vi "Undersample_NB.vi"(6 "error in (no error)":errorcluster, 7 "Unit Info":string="Unit1", 8 "U/S Frequency":i32=2400, 9 "U/S Location":string(combo)="VCO") -> (0 "error out":errorcluster, 2 "Cycle-Cycle Jitter":string, 3 "Total RMS Jitter":string)   [LabVIEW 2011]
doc: "This VI undersamples a selected signal from the NB PLL at a specified frequency.\n\nInputs:\n1. U/S Location: Part of PLL loop to be undersamles (VCO, PllOut, VCO_Z, Spine, etc).\n2. U/S Frequency: Frequency at which the PLL to be undersampled is running (2400, 2600, etc.)\n3. Unit Info: Information about the unit to attach to undersampling results file.\n\nOutputs:\n1. Total RMS Jitter: The total RMS Jitter as read from the resultspectrum file.\n2. Cycle-Cycle Jitter: The Cycle-Cycle Jitter as read from the result spectrum file."
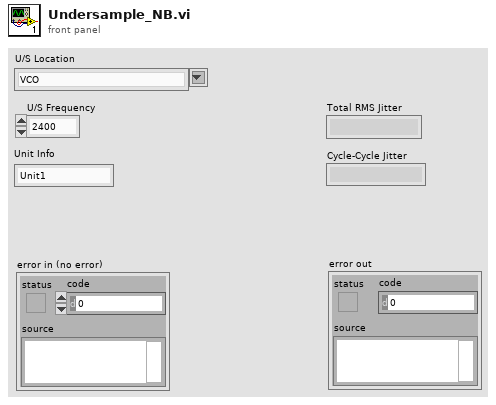
[diagram p1: front panel]
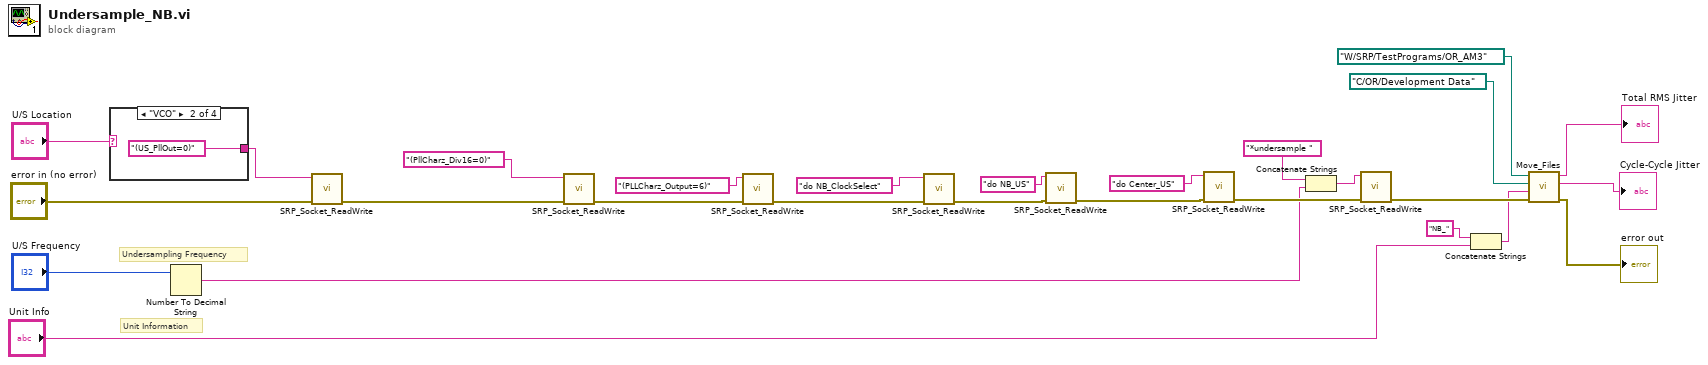
[diagram p0: block diagram]
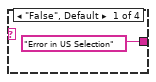
[diagram p2: hidden frame]
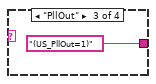
[diagram p3: hidden frame]
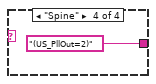
[diagram p4: hidden frame]
diagram:
  # "Unit Information"
  # "Undersampling Frequency"
  n1 = case shown="\"VCO\"" "U/S Location" {
    tunnel: ["Error in US Selection" "(US_PllOut=0)" "(US_PllOut=1)" "(US_PllOut=2)"] -> w10
    frame "False", Default {
    }
    frame "VCO" {
    }
    frame "PllOut" {
    }
    frame "Spine" {
    }
  }
  n2 = Number To Decimal String(number="U/S Frequency") -> (decimal integer string=w2:string)  [unwired: 1 in]
  n3 = call "SRP_Socket_ReadWrite.vi"("error in (no error)"="error in (no error)", "Data In"=w10) -> ("error out"=w24:errorcluster)  [unwired: 7 in, 1 out]
  n4 = call "SRP_Socket_ReadWrite.vi"("error in (no error)"=w24, "Data In"="(PllCharz_Div16=0)") -> ("error out"=w23:errorcluster)  [unwired: 7 in, 1 out]
  n5 = call "SRP_Socket_ReadWrite.vi"("error in (no error)"=w23, "Data In"="(PLLCharz_Output=6)") -> ("error out"=w22:errorcluster)  [unwired: 7 in, 1 out]
  n6 = call "SRP_Socket_ReadWrite.vi"("error in (no error)"=w22, "Data In"="do NB_ClockSelect") -> ("error out"=w19:errorcluster)  [unwired: 7 in, 1 out]
  n7 = call "SRP_Socket_ReadWrite.vi"("error in (no error)"=w19, "Data In"="do NB_US") -> ("error out"=w21:errorcluster)  [unwired: 7 in, 1 out]
  n8 = call "SRP_Socket_ReadWrite.vi"("error in (no error)"=w21, "Data In"="do Center_US") -> ("error out"=w20:errorcluster)  [unwired: 7 in, 1 out]
  n9 = Concatenate Strings("*undersample ", w2) -> (w4:string)
  n10 = call "SRP_Socket_ReadWrite.vi"("error in (no error)"=w20, "Data In"=w4) -> ("error out"=w17:errorcluster)  [unwired: 7 in, 1 out]
  n11 = Concatenate Strings("NB_" ("string"), "Unit Info") -> (w14:string)
  n12 = call "Move_Files.vi"("error in"=w17, "Unit Information"=w14, "Target Directory to Save U/S Files"=path "C:/OR/Development Data", "Location of U/S Files"=path "W:/SRP/TestPrograms/OR_AM3") -> ("error out"=→"error out":errorcluster, "Cycle-Cycle-Jitter"=→"Cycle-Cycle Jitter":string, "Total RMS Jitter"=→"Total RMS Jitter":string)  [unwired: 5 in]
